vi "VG_VerifTests_ModeRetour.vi"() -> ()   [LabVIEW 2020]
panel:
  out "Verification des tests en mode retour?":bool
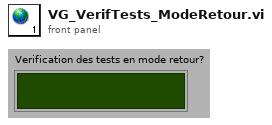
[diagram p1: front panel]
diagram:
